vi "StahlPS_Pbus.UpdateVoltage.vi"(0 "i ref in":refnum<vi>, 1 "badValue":bool, 2 "moduleValue":dbl format="%.2f", 3 "ms timeout (10000)":i32=10000, 4 "channelNumber":i32, 5 "error in (no error)":errorcluster, 6 "voltageQuality":i32) -> (14 "i ref out":refnum<vi>, 17 "timed out":bool, 19 "error out":errorcluster)   [LabVIEW 2014, in "StahlPS_Pbus.lvlib"]
doc: "Takes the inpute (raw) voltage and calcutes the real actual voltage [V] delivered by the power supply.\n\nThe value of the actual voltage is written to the attribute data and published via DIM.\n\nThe bad-status bit is also determined and updated."
uses:
  StahlPS_Pbus.lvlib
  CSlibraries/UtilityLib/UtilityLib.valueStatus.ctl
  CSCore/CSApplicationBaseClasses/PSChannelBase/PSChannelBase.directionType.ctl
  CSCore/CSApplicationBaseClasses/PSChannelBase/PSChannelBase.serviceType.ctl
  CSCore/CSApplicationBaseClasses/DeviceBase/DeviceBase.deviceState.ctl
  CSCore/CSApplicationBaseClasses/PSChannelBase/PSChannelBase.lvlib
  CSlibraries/UtilityLib/UtilityLib.lvlib
  CSCore/CSApplicationBaseClasses/DeviceBase/DeviceBase.lvlib
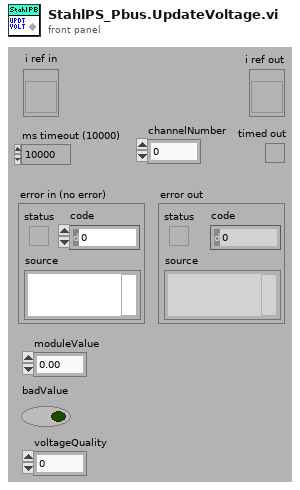
[diagram p1: front panel]
types:
  T1 = typedef "PSChannelBase.lvlib/PSChannelBase.serviceType.ctl" = enum16{"onOff", "voltage", "current", "tripCurrent", "rampUpSpeed", "rampDownSpeed", "status"}
  T2 = typedef "PSChannelBase.lvlib/PSChannelBase.directionType.ctl" = enum16{"unknown", "update actual value", "update nominal value", "update both"}
  T3 = typedef "UtilityLib.lvlib/UtilityLib.valueStatus.ctl" = enum16{"no info available", "stand by/off", "on", "warning", "alarm/malfunction", "not implemented", "user action required", "important information", "system default", "control default", "indicator default", "button default"}
  T4 = typedef "DeviceBase.lvlib/DeviceBase.deviceState.ctl" = i16
  T5 = typedef "StahlPS_Pbus.lvlib/StahlPS_Pbus.i attribute.ctl" = cluster{"Type":string, "CALC_FACTOR_SET_VOLTAGE":dbl, "CALC_FACTOR_GET_VOLTAGE":dbl, "CALC_FACTOR_GET_CURRENT":dbl, "CALC_FACTOR_SET_CURRENT ":dbl, "REG_VALUE":dbl, "Sign":bool, "setVoltIDs":i32[], "Elektrode Names":string[]}
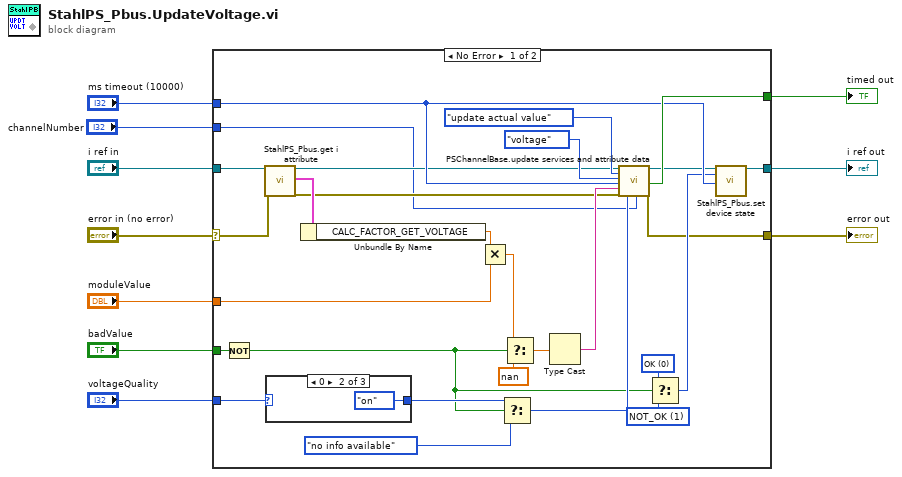
[diagram p0: block diagram]
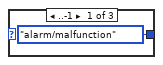
[diagram p2: hidden frame]
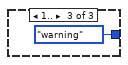
[diagram p3: hidden frame]
diagram:
  n1 = case shown="No Error" "error in (no error)" {
    selector: "error in (no error)" -> [w28 w42]
    tunnel: "i ref in" -> [w29 w43]
    tunnel: "moduleValue" -> [w26 _]
    tunnel: "ms timeout (10000)" -> [w20 _]
    tunnel: [w21 w43] -> w7
    tunnel: [w14 w42] -> w6
    tunnel: [w23 _] -> w5
    tunnel: "badValue" -> [w38 _]
    tunnel: "voltageQuality" -> [w37 _]
    tunnel: "channelNumber" -> [w11 _]
    frame No Error {
      w19 = T4 1 items=["ERROR"=-1, "OK"=0, "NOT_OK"=1] ("f")
      w18 = T4 0 items=["ERROR"=-1, "OK"=0, "NOT_OK"=1] ("deviceState")
      n2 = Not(x=w38) -> (.not. x?=w17:bool)
      n3 = call "StahlPS_Pbus.get i attribute.vi"("i ref in"=w29, "error in (no error)"=w28) -> ("i ref out"=w13:refnum<vi>, "i attribute"=w27:T5, "error out"=w12:errorcluster)  [unwired: 15 in]
      n4 = case shown="0" w37 {
        tunnel: [UtilityLib.valueStatus."alarm/malfunction" ("quality") UtilityLib.valueStatus."on" ("quality") UtilityLib.valueStatus."warning" ("quality")] -> w36
        frame ..-1 {
        }
        frame 0 {
        }
        frame 1.. {
        }
      }
      n5 = Unbundle By Name(w27) -> ("CALC_FACTOR_GET_VOLTAGE"=w30:dbl)
      n6 = Multiply(x=w30, y=w26) -> (x*y=w24:dbl)
      n7 = Select(t=w36, s=w17, f=UtilityLib.valueStatus."no info available" ("quality")) -> (s? t:f=w31:T3)
      n8 = Select(t=w24, s=w17, f=nan) -> (s? t:f=w33:dbl)
      n9 = Type Cast(x=w33) -> (*(type *) &x=w32:string)  [unwired: 1 in]
      n10 = call "PSChannelBase.update services and attribute data.vi"("i ref in"=w13, "direction"=PSChannelBase.directionType."update actual value", "service"=PSChannelBase.serviceType."voltage", "ms timeout (10000)"=w20, "value"=w32, "error in (no error)"=w12, "quality"=w31, "channelNumber"=w11) -> ("i ref out"=w15:refnum<vi>, "timed out"=w23:bool, "error out"=w14:errorcluster)  [unwired: 9 in]
      n11 = Select(t=w18, s=w17, f=w19) -> (s? t:f=w16:T4)
      n12 = call "StahlPS_Pbus.set device state.vi"("i ref in"=w15, "deviceState"=w16, "ms timeout (10000)"=w20) -> ("i ref out"=w21:refnum<vi>)  [unwired: 14 in, 2 out]
    }
    frame Error {
    }
  }
  "error out" <- w6
  "i ref out" <- w7
  "timed out" <- w5
